vi "VPI Init PWM.vi"(9 "pInitConfig":T1, 10 "DevIndex":i32, 11 "DevType":i32) -> (1 "pInitConfig out":T1, 3 "function return":i32)   [LabVIEW 2010, in "ControlPWM.lvlib"]
doc: "int WINAPI VPI_InitPWM(int DevType, int DevIndex, PVPI_INIT_CONFIG pInitConfig);"
uses:
  ControlPWM.lvlib
  ControlPWM/Ginkgo_Driver.dll
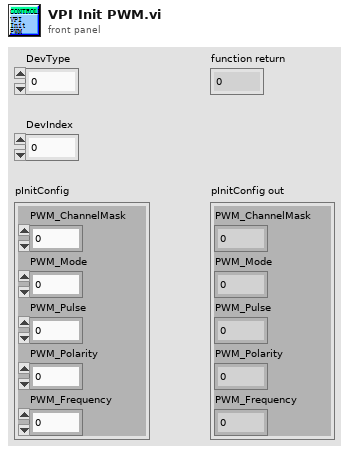
[diagram p1: front panel]
types:
  T1 = cluster{"PWM_ChannelMask":u8, "PWM_Mode":u8, "PWM_Pulse":u8, "PWM_Polarity":u8, "PWM_Frequency":u32}
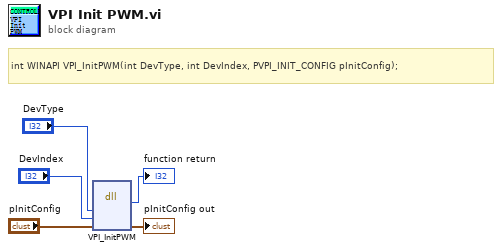
[diagram p0: block diagram]
diagram:
  # "int WINAPI VPI_InitPWM(int DevType, int DevIndex, PVPI_INIT_CONFIG pInitConfig);"
  n1 = dll-call lib="E:/Project/vt_ginkgo/truck/Ginkgo Driver/vs2010/Ginkgo_USB-I2C&SPI&CAN_API_v2.0.3.3/lib/labview_32bit/ControlPWM/Ginkgo_Driver.*" fn="VPI_InitPWM"("DevType"="DevType", "DevIndex"="DevIndex", "pInitConfig"="pInitConfig") -> (→"function return":i32, "pInitConfig"=→"pInitConfig out":T1)  [unwired: 5 in, 2 out]
